vi "Load Cfg.vi"(8 "error in (no error)":errorcluster, 11 "Communication Channel in":refnum<class "Communication Channel.lvclass">) -> (0 "error out":errorcluster, 3 "Communication Channel out":refnum<class "Communication Channel.lvclass">)   [LabVIEW 2018, in "Communication Channel.lvclass"]
uses:
  Communication Channel.lvclass
  Communication Channel.lvclass/Communication Channel.ctl
  <vilib>/Utility/config.llb/Read Key (String).vi
  <vilib>/Utility/config.llb/Read Key (U32).vi
  Socket2/Socket2/Socket2.lvclass
  RxTx/RxTx.lvclass
  <vilib>/Utility/config.llb/NI_LVConfig.lvlib
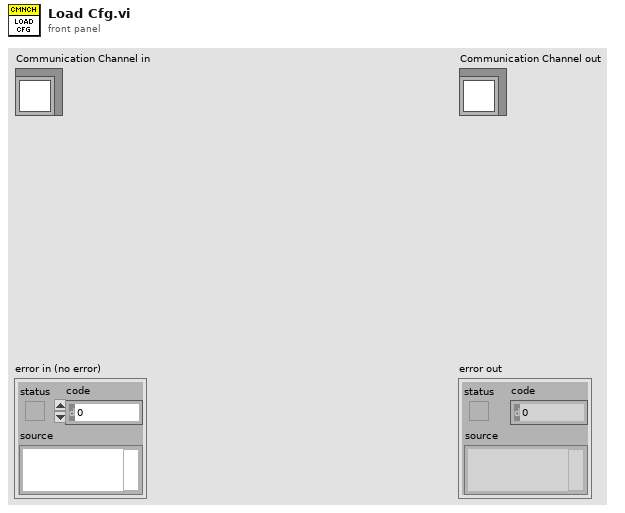
[diagram p1: front panel]
types:
  T1 = typedef "NI_LVConfig.lvlib/Config Data RefNum.ctl" = refnum<k1>
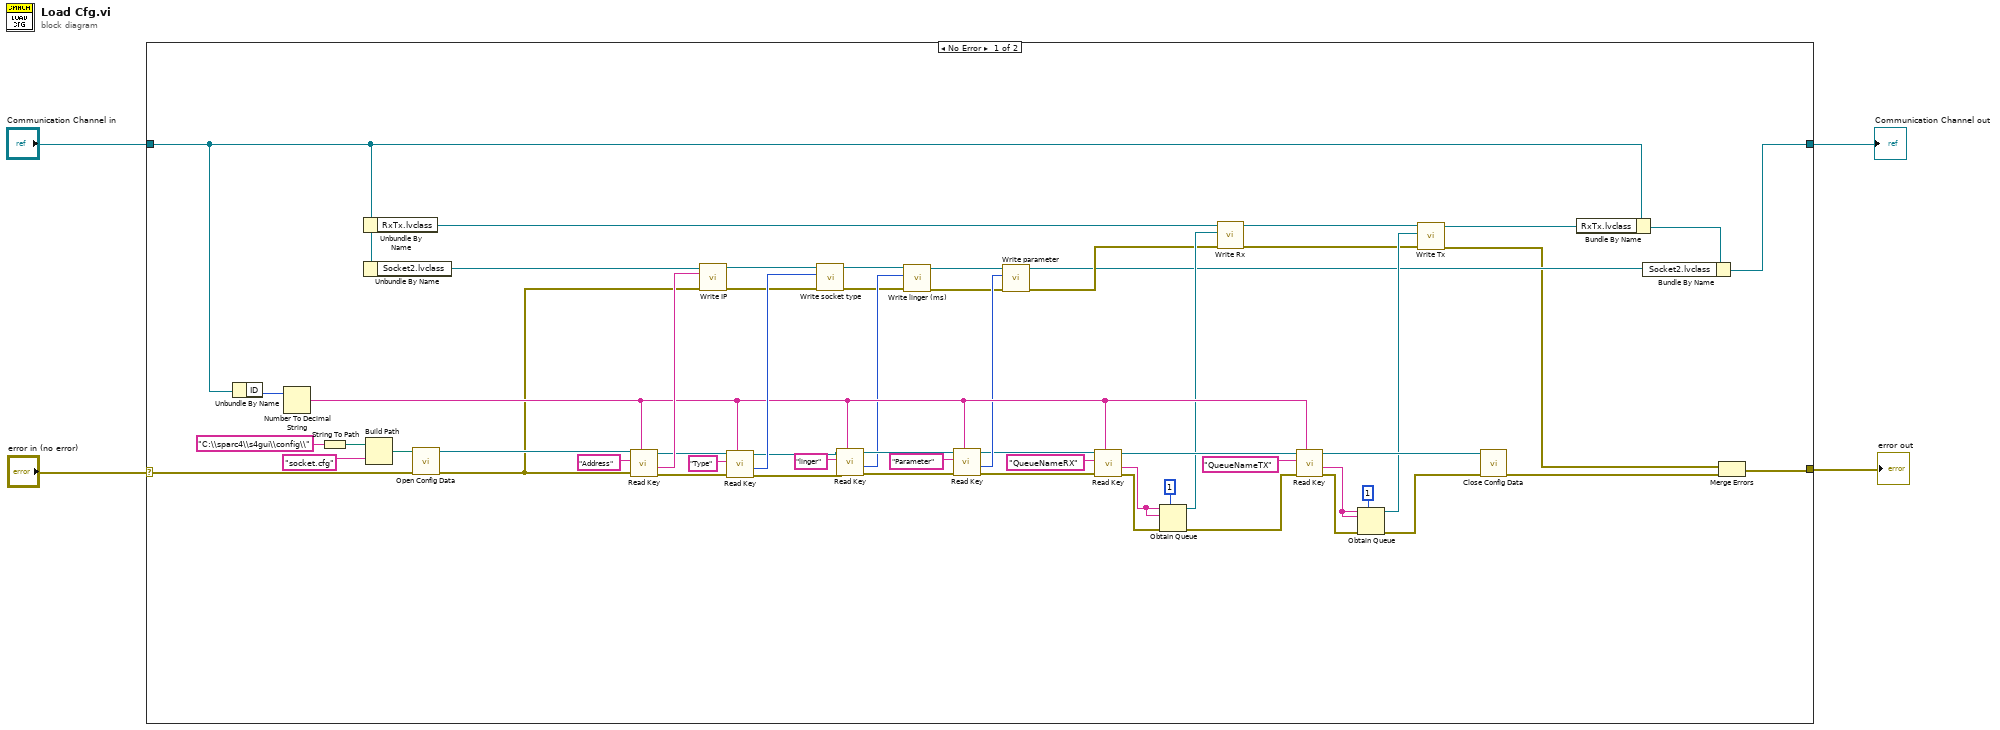
[diagram p0: block diagram]
diagram:
  n1 = case shown="No Error" "error in (no error)" {
    selector: "error in (no error)" -> [w19 w64]
    tunnel: [w6 w64] -> w3
    tunnel: [w9 w63] -> w1
    tunnel: "Communication Channel in" -> [w14 w63]
    frame No Error {
      n2 = Unbundle By Name(w14) -> ("ID"=w49:u32)
      n3 = Number To Decimal String(number=w49) -> (decimal integer string=w33:string)  [unwired: 1 in]
      n4 = String To Path(string="C:\\sparc4\\s4gui\\config\\" ("name or relative path")) -> (path=w46:path)
      n5 = Unbundle By Name(w14) -> ("RxTx.lvclass"=w18:refnum<class "RxTx.lvclass">)
      n6 = Unbundle By Name(w14) -> ("Socket2.lvclass"=w13:refnum<class "Socket2.lvclass">)
      n7 = Build Path(base path=w46, name or relative path="socket.cfg") -> (appended path=w62:path)
      n8 = call <vilib>:"Open Config Data.vi"("error in (no error)"=w19, "configuration file path"=w62) -> ("error out"=w5:errorcluster, "refnum"=w48:T1)  [unwired: 7 in, 1 out]
      n9 = call-poly <vilib>:"Read Key.vi"("section"=w33, "error in (no error)"=w5, "key"="Address", "refnum"=w48) -> ("error out"=w23:errorcluster, "value"=w40:string, "refnum out"=w36:T1)  [unwired: 4 in, 1 out]
      n10 = call-dynamic "Write IP.vi"("error in (no error)"=w5, "IP"=w40, "Socket in"=w13) -> ("error out"=w38:errorcluster, "Socket out"=w37:refnum<class "Socket2.lvclass">)  [unwired: 7 in]
      n11 = call-poly <vilib>:"Read Key.vi"("section"=w33, "error in (no error)"=w23, "key"="Type", "refnum"=w36) -> ("error out"=w22:errorcluster, "value"=w39:u32, "refnum out"=w35:T1)  [unwired: 4 in, 1 out]
      n12 = call-dynamic "Write socket type.vi"("error in (no error)"=w38, "Socket type"=w39, "Socket in"=w37) -> ("error out"=w31:errorcluster, "Socket out"=w30:refnum<class "Socket2.lvclass">)  [unwired: 7 in]
      n13 = call-poly <vilib>:"Read Key.vi"("section"=w33, "error in (no error)"=w22, "key"="linger", "refnum"=w35) -> ("error out"=w21:errorcluster, "value"=w32:u32, "refnum out"=w34:T1)  [unwired: 4 in, 1 out]
      n14 = call-dynamic "Write linger (ms).vi"("error in (no error)"=w31, "linger (ms)"=w32, "Socket in"=w30) -> ("error out"=w28:errorcluster, "Socket out"=w27:refnum<class "Socket2.lvclass">)  [unwired: 7 in]
      n15 = call-poly <vilib>:"Read Key.vi"("section"=w33, "error in (no error)"=w21, "key"="Parameter", "refnum"=w34) -> ("error out"=w20:errorcluster, "value"=w29:u32, "refnum out"=w24:T1)  [unwired: 4 in, 1 out]
      n16 = call-dynamic "Write parameter.vi"("error in (no error)"=w28, "Socket option"=w29, "Socket2 in"=w27) -> ("error out"=w17:errorcluster, "Socket2 out"=w12:refnum<class "Socket2.lvclass">)  [unwired: 7 in]
      n17 = call-poly <vilib>:"Read Key.vi"("section"=w33, "error in (no error)"=w20, "key"="QueueNameRX", "refnum"=w24) -> ("error out"=w53:errorcluster, "value"=w59:string, "refnum out"=w58:T1)  [unwired: 4 in, 1 out]
      n18 = Obtain Queue(max queue size (-1, unlimited)=1, name (unnamed)=w59, element data type=w59, error in (no error)=w53) -> (queue out=w26:refnum<queue>, error out=w52:errorcluster)  [unwired: 1 in, 1 out]
      n19 = call-dynamic "Write Rx.vi"("error in (no error)"=w17, "Rx"=w26, "RxTx in"=w18) -> ("error out"=w16:errorcluster, "RxTx out"=w15:refnum<class "RxTx.lvclass">)  [unwired: 7 in]
      n20 = call-poly <vilib>:"Read Key.vi"("section"=w33, "error in (no error)"=w52, "key"="QueueNameTX", "refnum"=w58) -> ("error out"=w51:errorcluster, "value"=w60:string, "refnum out"=w45:T1)  [unwired: 4 in, 1 out]
      n21 = Obtain Queue(max queue size (-1, unlimited)=1, name (unnamed)=w60, element data type=w60, error in (no error)=w51) -> (queue out=w25:refnum<queue>, error out=w44:errorcluster)  [unwired: 1 in, 1 out]
      n22 = call-dynamic "Write Tx.vi"("error in (no error)"=w16, "Tx"=w25, "RxTx in"=w15) -> ("error out"=w8:errorcluster, "RxTx out"=w10:refnum<class "RxTx.lvclass">)  [unwired: 7 in]
      n23 = call <vilib>:"Close Config Data.vi"("error in (no error)"=w44, "refnum"=w45) -> ("error out"=w7:errorcluster)  [unwired: 8 in, 1 out]
      n24 = Bundle By Name(cluster=w14, "RxTx.lvclass"=w10) -> (w11:refnum<class "Communication Channel.lvclass">)
      n25 = Bundle By Name(cluster=w11, "Socket2.lvclass"=w12) -> (w9:refnum<class "Communication Channel.lvclass">)
      n26 = Merge Errors(w8, w7) -> (w6:errorcluster)
    }
    frame Error {
    }
  }
  "error out" <- w3
  "Communication Channel out" <- w1
